vi "Complex Queue PtByPt.vi"(6 "initial queue element":cdb, 7 "initialize":bool, 10 "sample length":i32=100, 11 "input data point":cdb format="%#.6g") -> (0 "error":i32, 1 "Previous Queue":cdb[](array[numeric]), 2 "Current Queue":cdb[](array[numeric]), 3 "eliminated element":cdb format="%#.6g", 4 "current length":i32)   [LabVIEW 2017, in "NI_PtbyPt.lvlib"]
doc: "Creates a data queue of complex numbers."
uses:
  <vilib>/ptbypt/NI_PtbyPt.lvlib
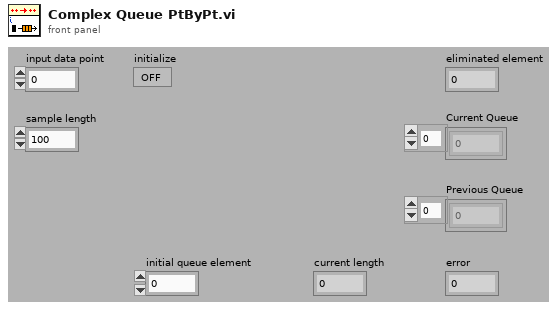
[diagram p1: front panel]
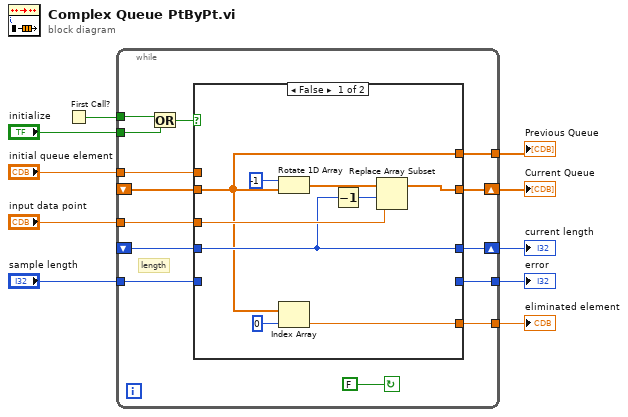
[diagram p0: block diagram]
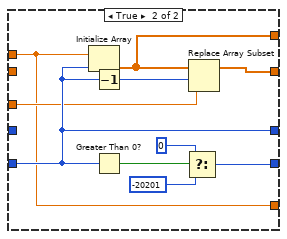
[diagram p2: hidden frame]
diagram:
  n1 = First Call?() -> (First Call?: T/F=w8:bool)
  n2 = while {
    tunnel: [w17] -> w7
    tunnel: w8 -> [w18]
    shift-left: _ -> [w22]
    shift-right: [w23] -> w9
    shift-left: _ -> [w21]
    shift-right: [w24] -> w10
    tunnel: "input data point" -> [w16]
    tunnel: "initialize" -> [w15]
    tunnel: "sample length" -> [w14]
    tunnel: "initial queue element" -> [w13]
    tunnel: [w12] -> w2
    tunnel: [w11] -> w1
    stop <- FALSE continue-if-true
    # "length"
    n3 = Or(x=w18, y=w15) -> (x .or. y?=w19:bool)
    n4 = case shown="False" w19 {
      tunnel: [w30 w43] -> w24
      tunnel: [w31 w39] -> w23
      tunnel: w22 -> [w31 _]
      tunnel: w21 -> [w27 _]
      tunnel: w16 -> [w32 w36]
      tunnel: [w27 w38] -> w17
      tunnel: w14 -> [_ w39]
      tunnel: w13 -> [_ w34]
      tunnel: [_ w35] -> w12
      tunnel: [w25 w34] -> w11
      frame False {
        n5 = Rotate 1D Array(1:w27, 2:i16 -1 ("n")) -> (0:w28:cdb[])
        n6 = Index Array(array=w27, index=0 ("Index")) -> (element=w25:cdb)
        n7 = Decrement(x=w31) -> (x-1=w29:i32)
        n8 = Replace Array Subset(array=w28, new element=w32, index=w29) -> (w30:cdb[])
      }
      frame True {
        n9 = Initialize Array(w34, w39) -> (w38:cdb[])
        n10 = Decrement(x=w39) -> (x-1=w37:i32)
        n11 = Greater Than 0?(x=w39) -> (x > 0?=w42:bool)
        n12 = Select(t=0, s=w42, f=-20201) -> (s? t:f=w35:i32)
        n13 = Replace Array Subset(array=w38, new element=w36, index=w37) -> (w43:cdb[])
      }
    }
  }
  "Current Queue" <- w10
  "current length" <- w9
  "Previous Queue" <- w7
  "error" <- w2
  "eliminated element" <- w1
